vi "EXOLABVIEW.vi"   [LabVIEW 2010]
uses:
  act/lv_01/lv_01.lvlib
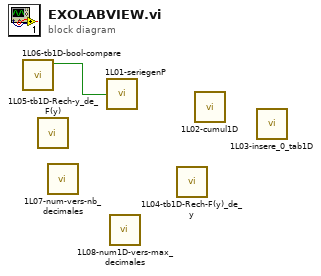
[diagram p0: block diagram]
diagram:
  n1 = call "1L06-tb1D-bool-compare.vi"() -> ("t1 <>t2 ?"=w1:bool)  [unwired: 11 in]
  n2 = call "1L05-tb1D-Rech-y_de_F(y).vi"() -> ()  [unwired: 3 in, 1 out]
  n3 = call "1L07-num-vers-nb_decimales.vi"() -> ()  [unwired: 11 in, 1 out]
  n4 = call "1L01-seriegenP.vi"("x_deb"=w1) -> ()  [unwired: 2 in, 1 out]
  n5 = call "1L08-num1D-vers-max_decimales.vi"() -> ()  [unwired: 1 in, 1 out]
  n6 = call "1L04-tb1D-Rech-F(y)_de_y.vi"() -> ()  [unwired: 3 in, 1 out]
  n7 = call "1L02-cumul1D.vi"() -> ()  [unwired: 4 in, 4 out]
  n8 = call "1L03-insere_0_tab1D.vi"() -> ()  [unwired: 2 in, 1 out]
